vi "LViradon (SubVI).vi"(9 "N_det":dbl=40.0, 10 "N_rot":dbl=40.0, 11 "2-D Array of Real":dbl[][](array[numeric])) -> (0 "error out":errorcluster, 2 "Recon":T1(plugin-control), 3 "Refnum out":T1(plugin-control))   [LabVIEW 2018]
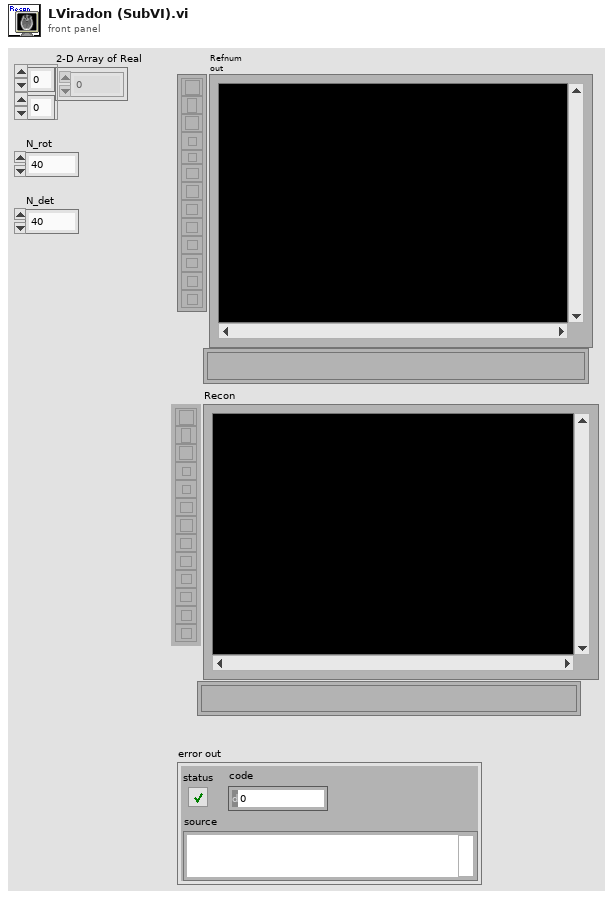
[diagram p1: front panel]
types:
  T1 = typedef "IMAQ Image.ctl" = refnum<image>
  T2 = typedef "Image Type" = u32
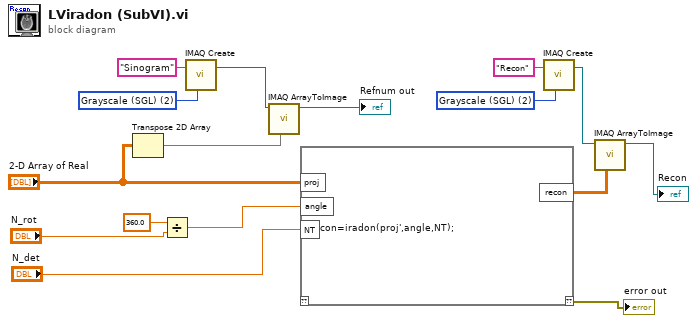
[diagram p0: block diagram]
diagram:
  w13 = T2 2 items=["Grayscale (U8)", "Grayscale (I16)", "Grayscale (SGL)", "Complex (CSG)", "RGB (U32)", "HSL (U32)", "RGB (U64)", "Grayscale (U16)"] ("Image Type")
  w10 = T2 2 items=["Grayscale (U8)", "Grayscale (I16)", "Grayscale (SGL)", "Complex (CSG)", "RGB (U32)", "HSL (U32)", "RGB (U64)", "Grayscale (U16)"] ("Image Type")
  n1 = Transpose 2D Array(2D array="2-D Array of Real") -> (transposed array=w1:dbl[][])
  n2 = Divide(x=360.0, y="N_rot") -> (x/y=w6:dbl)
  n3 = call "IMAQ Create"("Image Name"="Sinogram", "Image Type"=w10) -> ("New Image"=w11:T1)  [unwired: 3 in, 1 out]
  n4 = call "IMAQ ArrayToImage"("Image Pixels (Float)"=w1, "Image"=w11) -> ("Image Out"=→"Refnum out":T1)  [unwired: 8 in, 1 out]
  n5 = script code="recon=iradon(proj',angle,NT);"("proj"="2-D Array of Real", "angle"=w6, "NT"="N_det") -> ("??"=→"error out":errorcluster, "recon"=w15:dbl[][])  [unwired: 1 in]
  n6 = call "IMAQ Create"("Image Name"="Recon", "Image Type"=w13) -> ("New Image"=w14:T1)  [unwired: 3 in, 1 out]
  n7 = call "IMAQ ArrayToImage"("Image Pixels (Float)"=w15, "Image"=w14) -> ("Image Out"=→"Recon":T1)  [unwired: 8 in, 1 out]
